vi "WPI_DMAAddChannelToStream_AnalogTrigger.vi"(7 "AnalogTriggerDevRef":T1, 8 "error in (no error)":errorcluster, 10 "Analog Trigger Output Type":T3=enum."TriggerState", 11 "DMARef":T4) -> (0 "error out":errorcluster, 3 "DMARef":T4)   [LabVIEW 2017]
doc: "Specifies the data transferred in the DMA stream. Wire a device reference from the other WPI Robotics Library Open VIs to specify the data you want to receive. The order that the AddChannel VIs add data to the DMA stream defines the order that the Read VI returns the data.\n\nSpecifies the analog trigger data transferred in the DMA stream.\n\nYou must open a reference to a DMA stream with the Open VI before using this VI.\n\nThis software is licensed. Open the labview\\readme\\WPI Robotics Library Open Source License.txt file for more information."
uses:
  <vilib>/Rock Robotics/WPI/DMA/WPI_DMARef.ctl
  <vilib>/Rock Robotics/SystemInterfaces/AnalogTrigger/FPGA_AnalogTriggerStaticOutType.ctl
  <vilib>/Rock Robotics/SystemInterfaces/AnalogTrigger/FPGA_AnalogTriggerDevRef.ctl
  <vilib>/Rock Robotics/SystemInterfaces/AnalogTrigger/FPGA_AnalogTriggerIndex.ctl
  <vilib>/Rock Robotics/WPI/DMA/WPI_DMAChannelTypeEnum.ctl
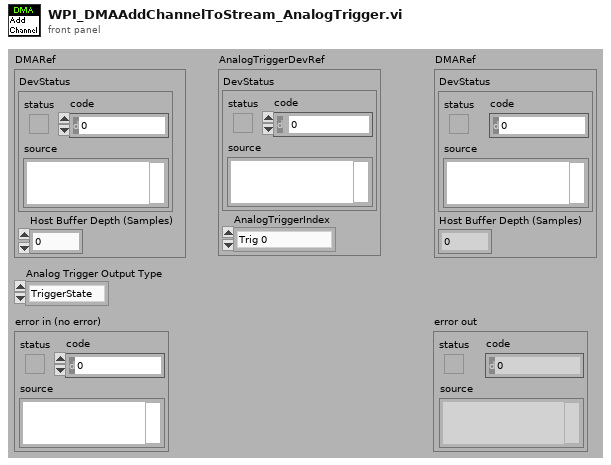
[diagram p1: front panel]
types:
  T1 = typedef "FPGA_AnalogTriggerDevRef.ctl" = cluster{"DevStatus":errorcluster, "AnalogTriggerIndex":T2}
  T2 = typedef "FPGA_AnalogTriggerIndex.ctl" = enum8{"Trig 0", "Trig 1", "Trig 2", "Trig 3", "Trig 4", "Trig 5", "Trig 6", "Trig 7", "Invalid"}
  T3 = typedef "FPGA_AnalogTriggerStaticOutType.ctl" = enum16{"InWindow", "TriggerState"}
  T4 = typedef "WPI_DMARef.ctl" = cluster{"DevStatus":errorcluster, "Host Buffer Depth (Samples)":u32}
  T5 = typedef "WPI_DMAChannelTypeEnum.ctl" = enum16{"AI (Raw)", "AI (Avg)", "Accumulator", "DI (Raw) Onboard", "DI (Filtered) Onboard", "DI (Raw) MXP", "DI (Filtered) MXP", "Analog Trigger", "Counter", "Counter (Timer)", "Encoder", "Encoder (Timer)", "Time Stamp"}
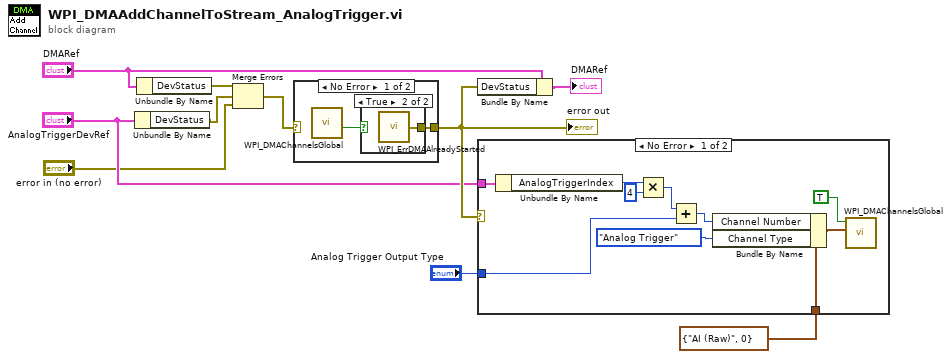
[diagram p0: block diagram]
diagram:
  n1 = Unbundle By Name("AnalogTriggerDevRef") -> ("DevStatus"=w3:errorcluster)
  n2 = Unbundle By Name("DMARef") -> ("DevStatus"=w4:errorcluster)
  n3 = Merge Errors(w4, w3, "error in (no error)") -> (w1:errorcluster)
  n4 = case shown="No Error" w1 {
    selector: w1 -> [_ w14]
    tunnel: [w11 w14] -> w9
    frame No Error {
      n5 = call <vilib>:"WPI_DMAChannelsGlobal.vi"() -> ("Started"=w12:bool)  [unwired: 4 in, 7 out]
      n6 = case shown="True" w12 {
        tunnel: [_ w13] -> w11
        frame False {
        }
        frame True {
          n7 = call <vilib>:"WPI_ErrDMAAlreadyStarted.vi"() -> ("error out"=w13:errorcluster)
        }
      }
    }
    frame Error {
    }
  }
  "error out" <- w9
  n8 = Bundle By Name(cluster="DMARef", "DevStatus"=w9) -> (→"DMARef":T4)
  n9 = case shown="No Error" w9 {
    tunnel: "AnalogTriggerDevRef" -> [w23 _]
    tunnel: cluster{"Channel Type":T5, "Channel Number":u8} {"Channel Type"=enum."AI (Raw)", "Channel Number"=0} ("Channel") -> [w22 _]
    tunnel: "Analog Trigger Output Type" -> [w15 _]
    frame No Error {
      n10 = Unbundle By Name(w23) -> ("AnalogTriggerIndex"=w19:T2)
      n11 = Multiply(x=w19, y=4) -> (x*y=w17:i32)
      n12 = Add(x=w17, y=w15) -> (x+y=w16:i32)
      n13 = Bundle By Name(cluster=w22, "Channel Number"=w16, "Channel Type"=WPI_DMAChannelTypeEnum."Analog Trigger") -> (w21:cluster{"Channel Type":T5, "Channel Number":u8})
      n14 = call <vilib>:"WPI_DMAChannelsGlobal.vi"("Channel"=w21, "Add"=TRUE) -> ()  [unwired: 2 in, 8 out]
    }
    frame Error {
    }
  }
